vi "Apply Module Configuration Data.vi"(8 "Error In":errorcluster, 11 "Compiled.Settings":T1 {"Configuration Data"."Properties"."U64 Properties"."UInt64 Write" format="%.0x"; "Configuration Data"."Properties"."U32 Properties"."UInt32 Write" format="%.0x"; "Configuration Data"."Properties"."Double Properties"."Double Write" format="%_20g"}) -> (0 "Error Out":errorcluster, 2 "Device Session":refnum<k21>, 3 "SLSC Module Name":refnum<k21>)   [LabVIEW 2020, in "SLSC-12201 DIO Engine.lvlib"]
uses:
  SLSC-12201 DIO Engine.lvlib
  Shared/Compiled.Settings
  Shared/SLSC Dynamic Channel.ctl
  Shared/SLSC Dynamic Channel Type.ctl
  <vilib>/SLSC/Initialize Session with Devices.vi
  <vilib>/NI VeriStand/Custom Device Tools/Custom Device Utility Library/Custom Device Utility Library.lvlib
  <vilib>/NI VeriStand/Custom Device Tools/Custom Device Utility Library/RT Debug String Color Spec.ctl
  <vilib>/SLSC/SLSC.lvlib
  Shared/SLSC-12201 DIO Shared.lvlib
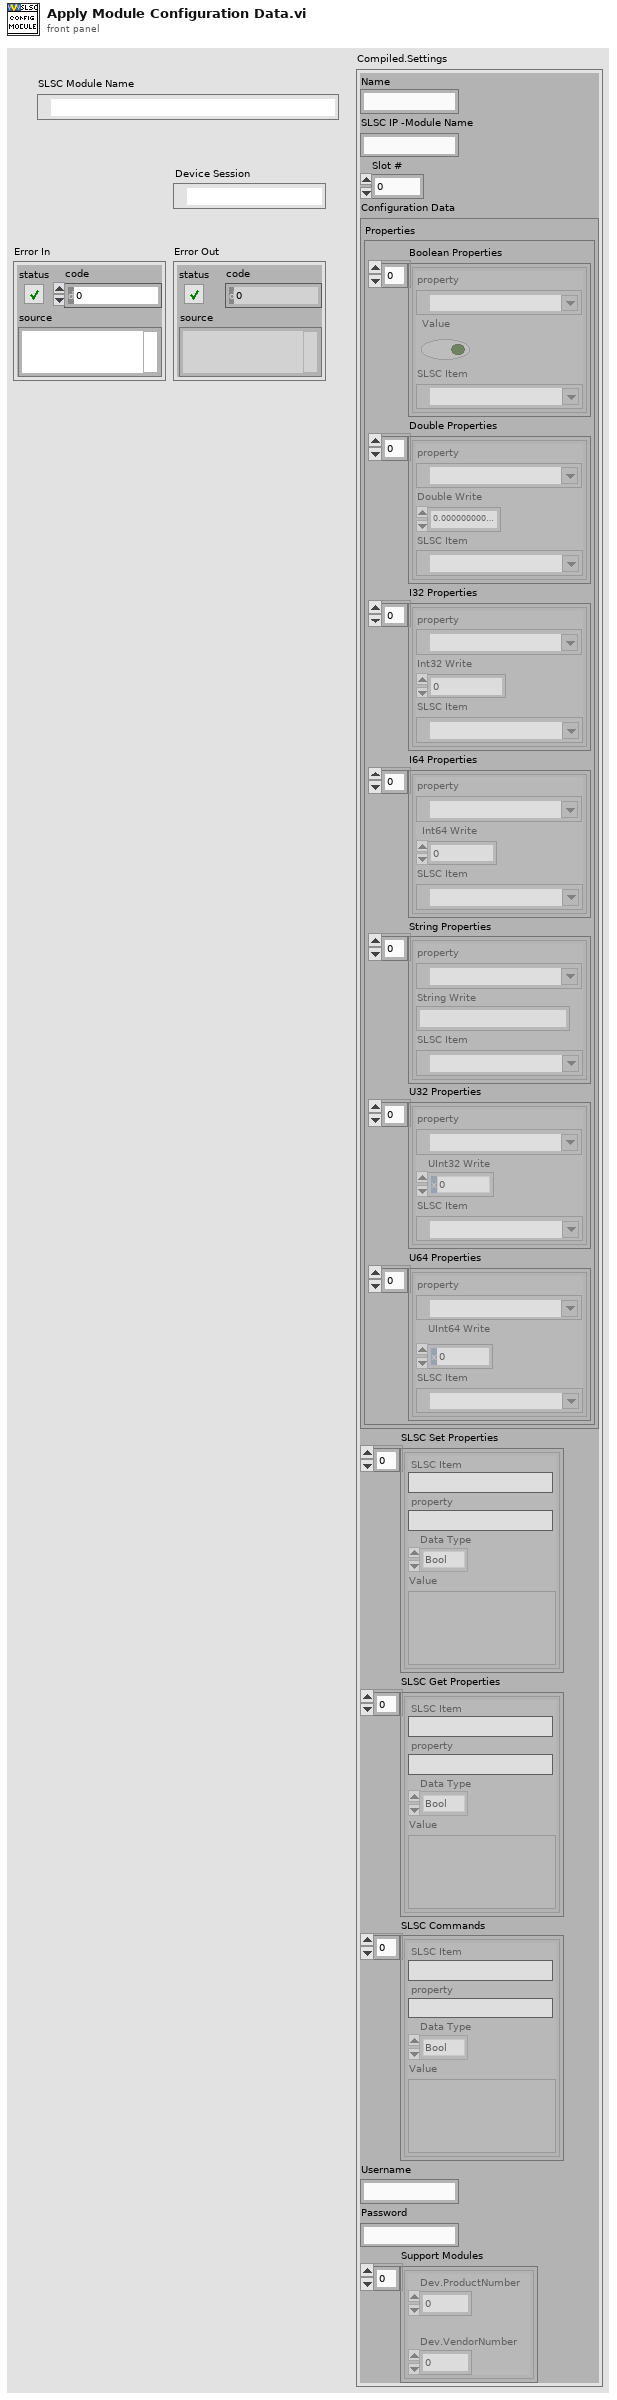
[diagram p1: front panel]
types:
  T1 = typedef "SLSC-12201 DIO Shared.lvlib/Compiled.Settings" = cluster{"Name":string, "SLSC IP -Module Name":string, "Slot #":i32, "Configuration Data":cluster{"Properties":cluster{"Boolean Properties":cluster{"property":refnum<k21>, "Value":bool, "SLSC Item":refnum<k21>}[], "Double Properties":cluster{"property":refnum<k21>, "Double Write":dbl, "SLSC Item":refnum<k21>}[], "I32 Properties":cluster{"property":refnum<k21>, "Int32 Write":i32, "SLSC Item":refnum<k21>}[], "I64 Properties":cluster{"property":refnum<k21>, "Int64 Write":i64, "SLSC Item":refnum<k21>}[], "String Properties":cluster{"property":refnum<k21>, "String Write":string, "SLSC Item":refnum<k21>}[], "U32 Properties":cluster{"property":refnum<k21>, "UInt32 Write":u32, "SLSC Item":refnum<k21>}[], "U64 Properties":cluster{"property":refnum<k21>, "UInt64 Write":u64, "SLSC Item":refnum<k21>}[]}}, "SLSC Set Properties":T2[], "SLSC Get Properties":T2[], "SLSC Commands":T2[], "Username":string, "Password":string, "Support Modules":cluster{"Dev.ProductNumber":u32, "Dev.VendorNumber":u32}[]}
  T2 = typedef "SLSC-12201 DIO Shared.lvlib/SLSC Dynamic Channel.ctl" = cluster{"SLSC Item":string, "property":string, "Data Type":T3, "Value":variant}
  T3 = typedef "SLSC-12201 DIO Shared.lvlib/SLSC Dynamic Channel Type.ctl" = enum16{"Bool", "Double", "I32", "I64", "String", "U32", "U64", "EnumI32"}
  T4 = typedef "Custom Device Utility Library.lvlib/RT Debug String Color Spec.ctl" = u16
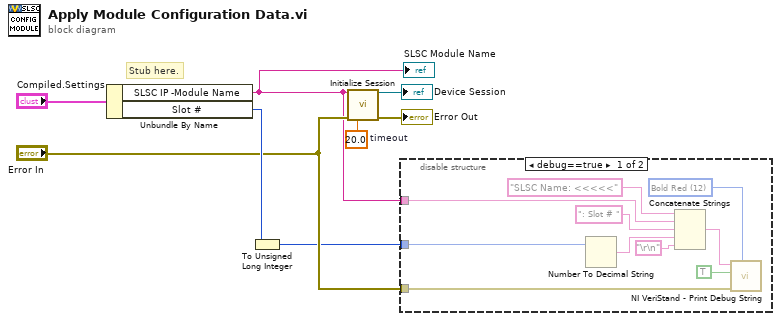
[diagram p0: block diagram]
diagram:
  w5 = 20.0  # timeout
  # "Stub here."
  n1 = Unbundle By Name("Compiled.Settings") -> ("SLSC IP -Module Name"=w3:string, "Slot #"=w7:i32)
  "SLSC Module Name" <- w3
  n2 = To Unsigned Long Integer(number=w7) -> (unsigned 32bit integer=w1:u32)
  n3 = call-poly <vilib>:"Initialize Session.vi"("devices"=w3, "error in (no error)"="Error In", "connect timeout (60 sec)"=w5) -> ("session out"=→"Device Session":refnum<k21>, "error out"=→"Error Out":errorcluster)  [unwired: 11 in]
  n4 = disable-structure shown="debug==true" {
    disable-tunnel: w3 -> [w18 _]
    disable-tunnel: "Error In" -> [w17 _]
    disable-tunnel: w1 -> [w10 _]
    frame condition #0 {
      w13 = T4 12 items=["Plain White"=7, "Bold White"=15, "Bold Blue"=9, "Bold Green"=10, "Bold Red"=12] ("Attribute")
      n5 = Number To Decimal String(number=w10) -> (decimal integer string=w9:string)  [unwired: 1 in]
      n6 = Concatenate Strings("SLSC Name: <<<<<" ("string"), w18, ": Slot # " ("string"), w9, "\r\n") -> (w16:string)
      n7 = call <vilib>:"NI VeriStand - Print Debug String.vi"("Attribute"=w13, "error in (no error)"=w17, "Add to log file? (F)"=TRUE ("Add to log file? (T)"), "Message"=w16) -> ()  [unwired: 7 in, 1 out]
    }
    frame condition #1 (active) {
    }
  }
